vi "geistest.vi"() -> ()   [LabVIEW 2025]
uses:
  PalmSens/PalmSens.lvclass
  C:/Users/stef/code/palmsenssdk/labview/PalmSens/Libraries/PalmSens.Core.Simplified.LabVIEW.dll
  PalmSens/Libraries/PalmSens.Core.Simplified.LabVIEW.dll
  PalmSens/MeasurementResults.ctl
  PalmSens/LiveCurveResult.ctl
panel:
  out "Results":T1
  out "Method Indicator":refnum<k24>
  out "Array":string[](array[string])
  out "Is Measuring":bool
  in  "PalmSens.lvclass":refnum<class "PalmSens.lvclass">
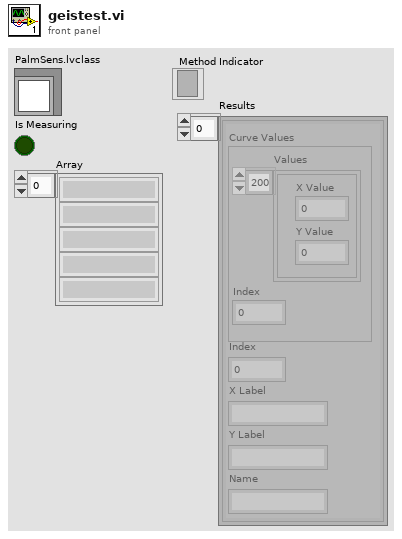
[diagram p1: front panel]
types:
  T1 = typedef "MeasurementResults.ctl" = T2[]
  T2 = typedef "LiveCurveResult.ctl" = cluster{"X Label":string, "Y Label":string, "Name":string, "Index":i16, "Curve Values":cluster{"Values":cluster{"X Value":dbl, "Y Value":dbl}[], "Index":i16}}
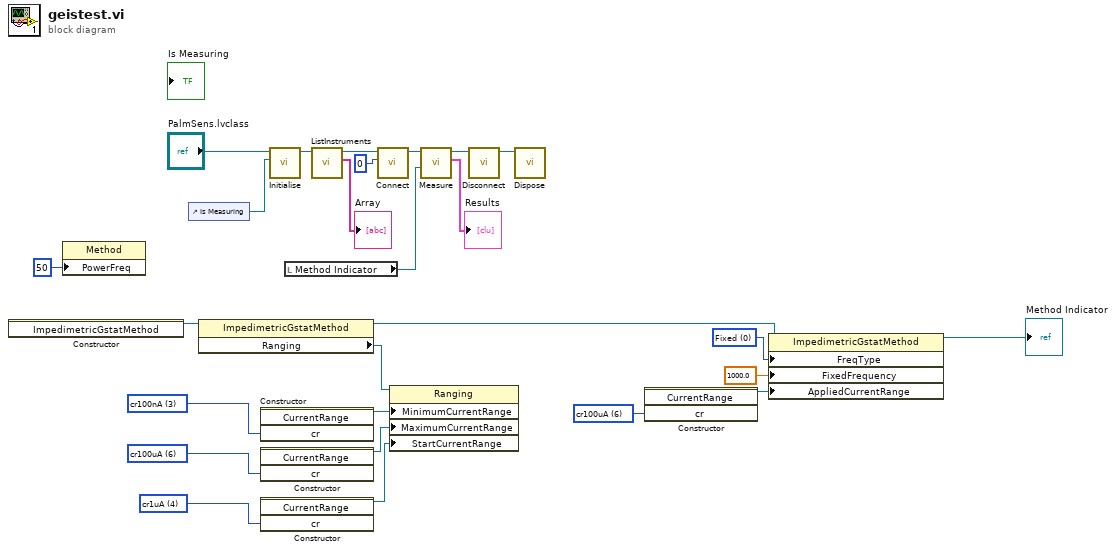
[diagram p0: block diagram]
diagram:
  w1 = 6 items=["cr100pA"=0, "cr1nA"=1, "cr10nA"=2, "cr100nA"=3, "cr1uA"=4, "cr10uA"=5, "cr100uA"=6, "cr1mA"=7, "cr10mA"=8, "cr100mA"=9, "cr2uA"=10, "cr4uA"=11, "cr8uA"=12, "cr16uA"=13, "cr32uA"=14, "cr125uA"=17, "cr250uA"=18, "cr500uA"=19, "cr5mA"=20, "cr6uA"=21, "cr13uA"=22, "cr25uA"=23, "cr50uA"=24, "cr200uA"=25, "cr63uA"=26, "cr1mA_shunt"=27, "cr10mA_shunt"=28, "cr100mA_shunt"=29, "cr1A"=30, "cr2500uA"=31] ("cr")
  w4 = 0 items=["Fixed", "Scan"] ("FreqType")
  w10 = 4 items=["cr100pA"=0, "cr1nA"=1, "cr10nA"=2, "cr100nA"=3, "cr1uA"=4, "cr10uA"=5, "cr100uA"=6, "cr1mA"=7, "cr10mA"=8, "cr100mA"=9, "cr2uA"=10, "cr4uA"=11, "cr8uA"=12, "cr16uA"=13, "cr32uA"=14, "cr125uA"=17, "cr250uA"=18, "cr500uA"=19, "cr5mA"=20, "cr6uA"=21, "cr13uA"=22, "cr25uA"=23, "cr50uA"=24, "cr200uA"=25, "cr63uA"=26] ("cr")
  w11 = 6 items=["cr100pA"=0, "cr1nA"=1, "cr10nA"=2, "cr100nA"=3, "cr1uA"=4, "cr10uA"=5, "cr100uA"=6, "cr1mA"=7, "cr10mA"=8, "cr100mA"=9, "cr2uA"=10, "cr4uA"=11, "cr8uA"=12, "cr16uA"=13, "cr32uA"=14, "cr125uA"=17, "cr250uA"=18, "cr500uA"=19, "cr5mA"=20, "cr6uA"=21, "cr13uA"=22, "cr25uA"=23, "cr50uA"=24, "cr200uA"=25, "cr63uA"=26] ("cr")
  w13 = 3 items=["cr100pA"=0, "cr1nA"=1, "cr10nA"=2, "cr100nA"=3, "cr1uA"=4, "cr10uA"=5, "cr100uA"=6, "cr1mA"=7, "cr10mA"=8, "cr100mA"=9, "cr2uA"=10, "cr4uA"=11, "cr8uA"=12, "cr16uA"=13, "cr32uA"=14, "cr125uA"=17, "cr250uA"=18, "cr500uA"=19, "cr5mA"=20, "cr6uA"=21, "cr13uA"=22, "cr25uA"=23, "cr50uA"=24, "cr200uA"=25, "cr63uA"=26] ("cr")
  n1 = constructor class="ImpedimetricGstatMethod"() -> (reference out=w20:refnum<k24>)  [unwired: 3 in, 2 out]
  n2 = property class="Method"("PowerFreq"=50) -> ()  [unwired: 2 in, 2 out]
  n3 = control-ref of="Is Measuring"() -> (w25:refnum<vi>)
  n4 = property class="ImpedimetricGstatMethod"(reference=w20) -> (reference out=w7:refnum<k24>, "Ranging"=w6:refnum<k24>)  [unwired: 1 in, 1 out]
  n5 = constructor class="CurrentRange"("cr"=w13) -> (reference out=w12:refnum<k24>)  [unwired: 3 in, 3 out]
  n6 = constructor class="CurrentRange"("cr"=w11) -> (reference out=w8:refnum<k24>)  [unwired: 3 in, 3 out]
  n7 = constructor class="CurrentRange"("cr"=w10) -> (reference out=w9:refnum<k24>)  [unwired: 3 in, 3 out]
  n8 = call-dynamic "Initialise.vi"("Is Measuring Refnum"=w25, "PalmSens in"="PalmSens.lvclass") -> ("PalmSens out"=w24:refnum<class "PalmSens.lvclass">)  [unwired: 8 in, 1 out]
  n9 = local read "Method Indicator"() -> (w14:refnum<k24>)
  n10 = call-dynamic "ListInstruments.vi"("PalmSens in"=w24) -> ("Array"=→"Array":string[], "PalmSens out"=w22:refnum<class "PalmSens.lvclass">)  [unwired: 8 in, 1 out]
  n11 = call-dynamic "Connect.vi"("Instrument Index"=0, "PalmSens in"=w22) -> ("PalmSens out"=w15:refnum<class "PalmSens.lvclass">)  [unwired: 8 in, 1 out]
  n12 = property class="Ranging"(reference=w6, "MinimumCurrentRange"=w12, "MaximumCurrentRange"=w8, "StartCurrentRange"=w9) -> ()  [unwired: 1 in, 2 out]
  n13 = call-dynamic "Measure.vi"("Method .NET Refnum"=w14, "PalmSens in"=w15) -> ("Curves"=→"Results":T1, "PalmSens out"=w16:refnum<class "PalmSens.lvclass">)  [unwired: 2 in, 2 out]
  n14 = call-dynamic "Disconnect.vi"("PalmSens in"=w16) -> ("PalmSens out"=w18:refnum<class "PalmSens.lvclass">)  [unwired: 9 in, 1 out]
  n15 = call-dynamic "Dispose.vi"("PalmSens in"=w18) -> ()  [unwired: 9 in, 2 out]
  n16 = constructor class="CurrentRange"("cr"=w1) -> (reference out=w2:refnum<k24>)  [unwired: 3 in, 3 out]
  n17 = property class="ImpedimetricGstatMethod"(reference=w7, "FreqType"=w4, "FixedFrequency"=sgl 1000.0, "AppliedCurrentRange"=w2) -> (reference out=→"Method Indicator":refnum<k24>)  [unwired: 1 in, 1 out]
